vi "index Uint in range.vi"(10 "limit":u8, 11 "index":u8) -> (3 "new index":u8)   [LabVIEW 2018]
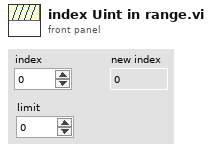
[diagram p1: front panel]
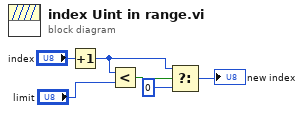
[diagram p0: block diagram]
diagram:
  n1 = Increment(x="index") -> (x+1=w4:u8)
  n2 = Less?(x=w4, y="limit") -> (x < y?=w5:bool)
  n3 = Select(t=w4, s=w5, f=u8 0) -> (s? t:f=→"new index":u8)
